vi "case selection.vi"(1 "Beamline Section":T1) -> (0 "VI Refnum":refnum<vi>)   [LabVIEW 2016, in "main.lvlib"]
uses:
  main.lvlib
  beamline selection.ctl
  controls/beamline sections.lvlib
  High energy end/High energy llb.lvlib
  low energy end/Low energy end/Low energy end llb.lvlib
  Transmission/transmission.lvlib
  R30/R30  library.lvlib
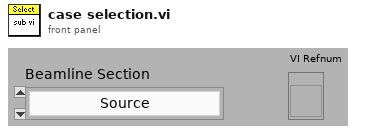
[diagram p1: front panel]
types:
  T1 = typedef "main.lvlib/beamline selection.ctl" = enum16{"Source", "Low End", "High End", "Transmission", "R30", "R45"}
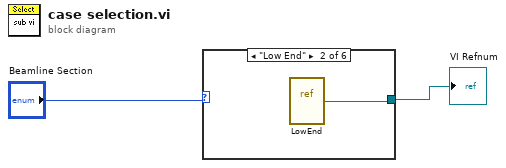
[diagram p0: block diagram]
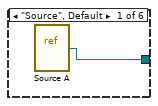
[diagram p2: hidden frame]
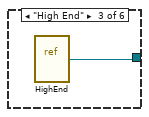
[diagram p3: hidden frame]
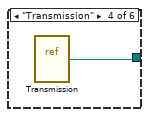
[diagram p4: hidden frame]
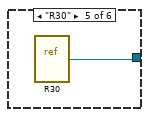
[diagram p5: hidden frame]
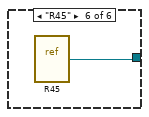
[diagram p6: hidden frame]
diagram:
  n1 = case shown="\"Low End\"" "Beamline Section" {
    tunnel: [w3 w4 w5 w6 w7 w8] -> w1
    frame "Source", Default {
      n2 = vi-ref "Source A.vi"() -> (w3:refnum<vi>)
    }
    frame "Low End" {
      n3 = vi-ref "LowEnd.vi"() -> (w4:refnum<vi>)
    }
    frame "High End" {
      n4 = vi-ref "HighEnd.vi"() -> (w5:refnum<vi>)
    }
    frame "Transmission" {
      n5 = vi-ref "Transmission.vi"() -> (w6:refnum<vi>)
    }
    frame "R30" {
      n6 = vi-ref "R30.vi"() -> (w7:refnum<vi>)
    }
    frame "R45" {
      n7 = vi-ref "R45.vi"() -> (w8:refnum<vi>)
    }
  }
  "VI Refnum" <- w1
